vi "Ball Align(SubVI).vi"(0 "Align X - t, Y - f":bool, 3 "x is in range":bool, 4 "y is in range":bool, 5 "L_PWM":dbl, 6 "R_PWM":dbl, 7 "curX":dbl, 8 "defY":dbl, 9 "curY":dbl, 14 "defX":dbl, 16 "Range":dbl) -> (13 "x_is_in_range":bool, 15 "y_is_in_range":bool, 20 "Align_X-t,Y-f":bool, 21 "Boolean 4":bool, 23 "Boolean":bool, 24 "Boolean 3":bool, 25 "Boolean 2":bool, 26 "L_PWM out":dbl, 27 "R_PWM out":dbl)   [LabVIEW 2017]
panel:
  in  "extra power":dbl format="%#_13g"
  in  "range for boost":dbl
  out "offset":bool
  in  "M_offsetX":dbl
  in  "M_defY":dbl
  # "IN"
  # "OUT"
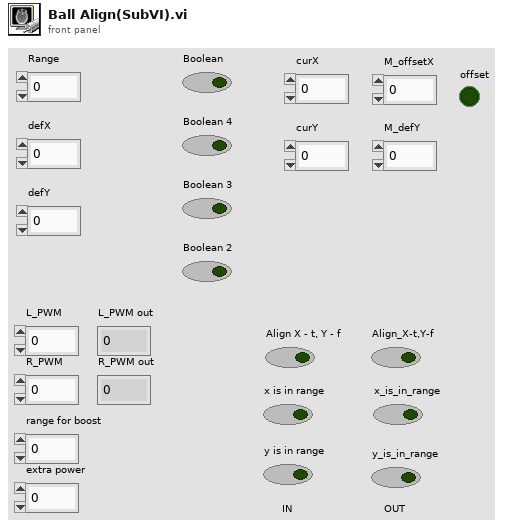
[diagram p1: front panel]
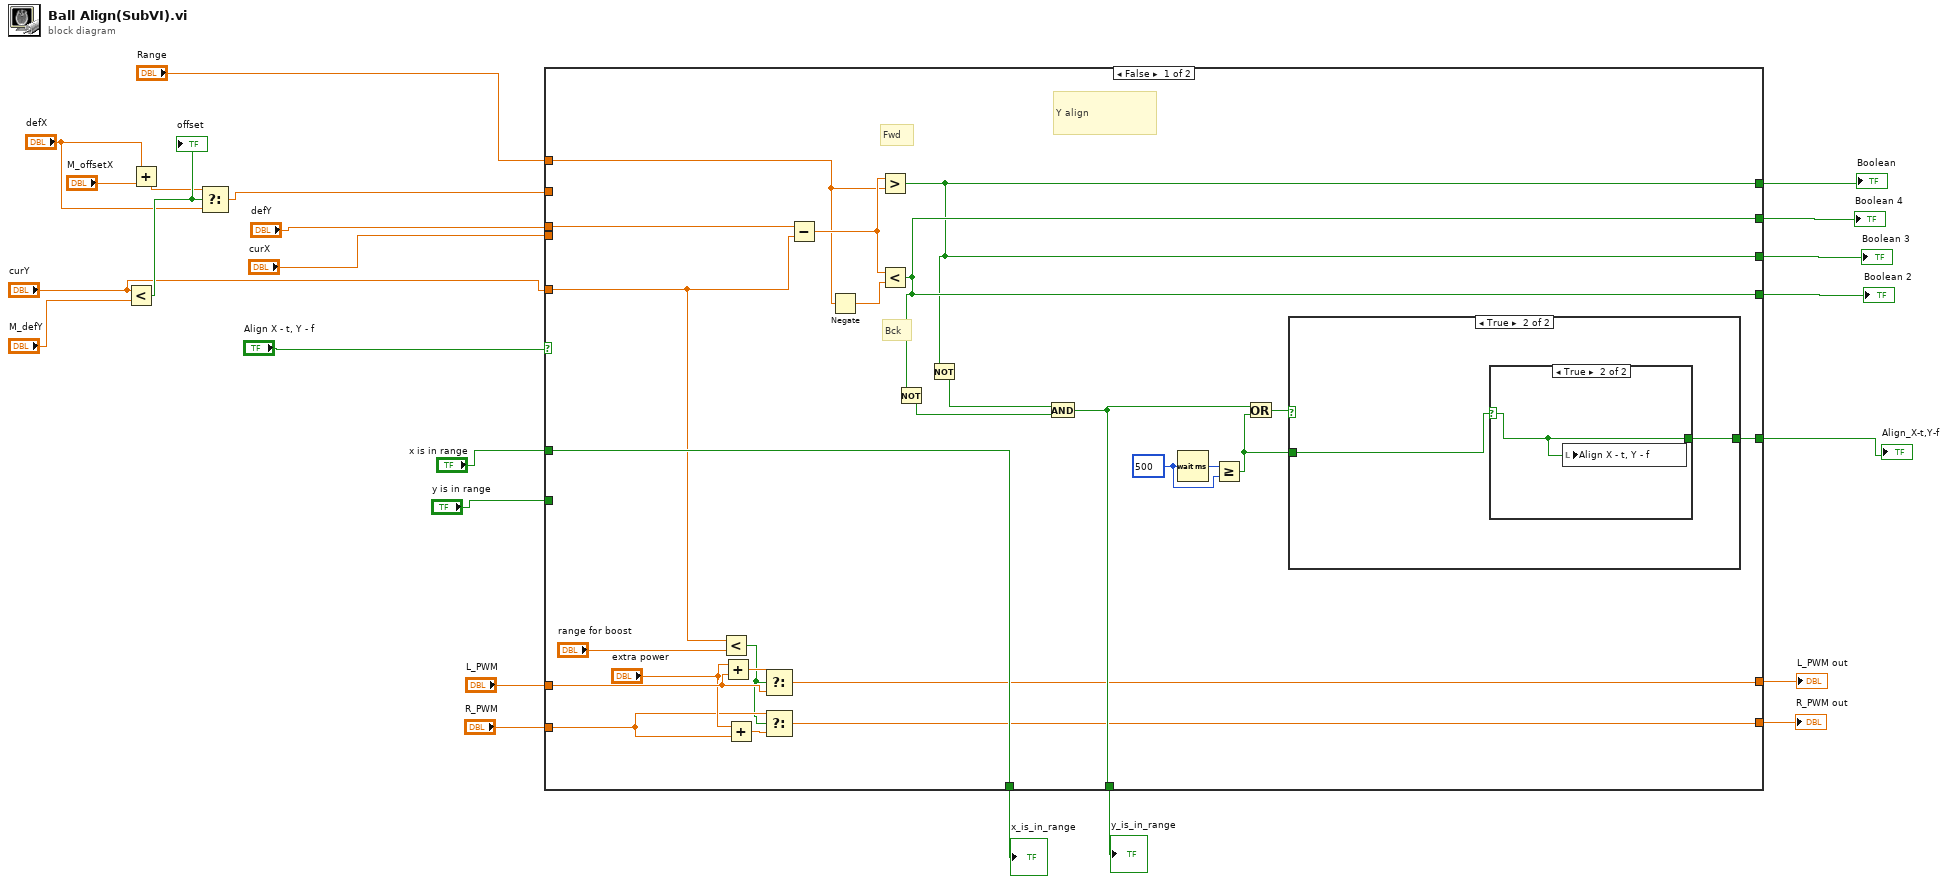
[diagram p0: block diagram]
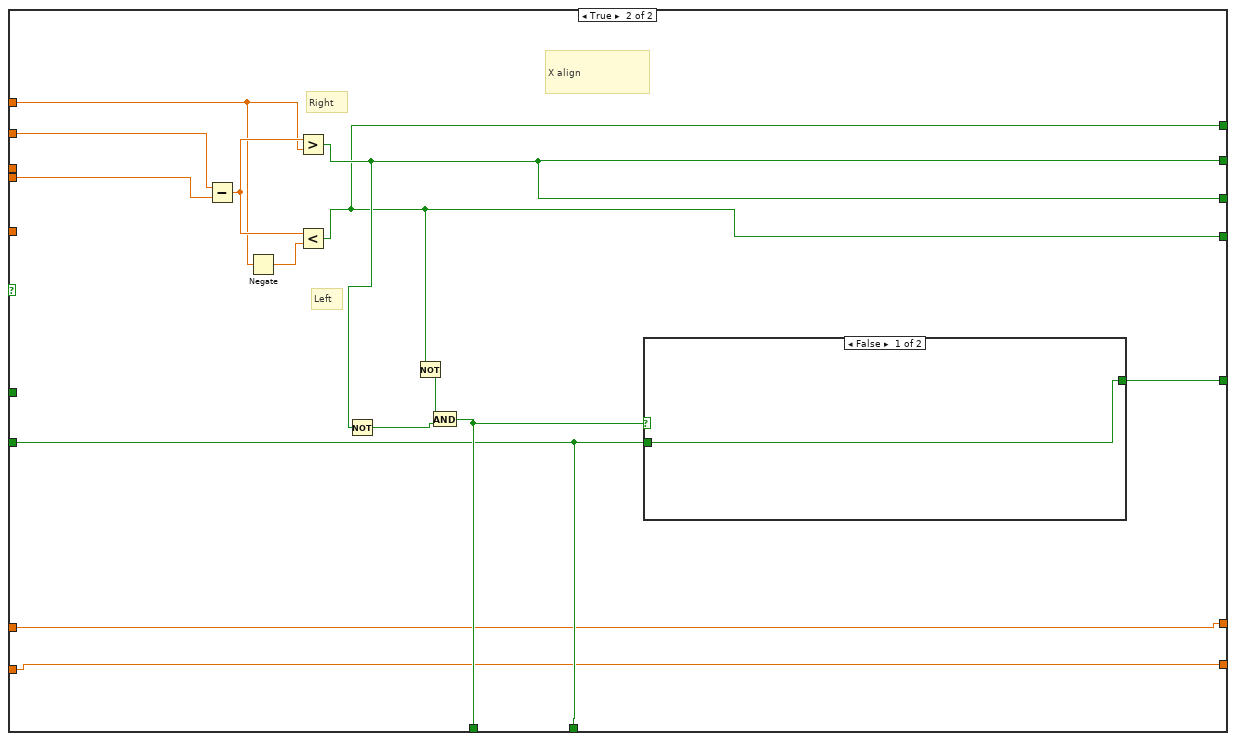
[diagram p4: hidden frame]
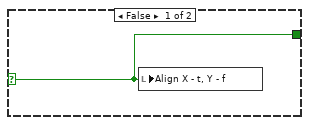
[diagram p6: hidden frame]
diagram:
  n1 = Less?(x="curY", y="M_defY") -> (x < y?=w13:bool)
  "offset" <- w13
  n2 = Add(x="defX", y="M_offsetX") -> (x+y=w11:dbl)
  n3 = Select(t=w11, s=w13, f="defX") -> (s? t:f=w9:dbl)
  n4 = case shown="False" "Align X - t, Y - f" {
    tunnel: w9 -> [_ w64]
    tunnel: "curX" -> [_ w63]
    tunnel: "Range" -> [w46 w62]
    tunnel: "defY" -> [w47 _]
    tunnel: "curY" -> [w34 _]
    tunnel: [w45 w58] -> w19
    tunnel: [w36 w61] -> w20
    tunnel: [w44 w60] -> w21
    tunnel: [w43 w60] -> w22
    tunnel: [w44 w59] -> w23
    tunnel: [w43 w59] -> w24
    tunnel: "x is in range" -> [w36 _]
    tunnel: "y is in range" -> [_ w58]
    tunnel: [w35 w57] -> w5
    tunnel: "L_PWM" -> [w31 w55]
    tunnel: "R_PWM" -> [w28 w56]
    tunnel: [w27 w55] -> w2
    tunnel: [w26 w56] -> w1
    frame False {
      w39 = u32 500 ("milliseconds to wait")
      # "Bck"
      # "Fwd"
      # "Y align"
      n5 = Less?(x=w34, y="range for boost") -> (x < y?=w25:bool)
      n6 = Add(x="extra power", y=w31) -> (x+y=w32:dbl)
      n7 = Add(x="extra power", y=w28) -> (x+y=w30:dbl)
      n8 = Select(t=w32, s=w25, f=w31) -> (s? t:f=w27:dbl)
      n9 = Select(t=w28, s=w25, f=w30) -> (s? t:f=w26:dbl)
      n10 = Subtract(x=w47, y=w34) -> (x-y=w49:dbl)
      n11 = Negate(x=w46) -> (-x=w48:dbl)
      n12 = Greater?(x=w49, y=w46) -> (0:w43:bool)
      n13 = Less?(x=w49, y=w48) -> (x < y?=w44:bool)
      n14 = Not(x=w44) -> (.not. x?=w41:bool)
      n15 = Not(x=w43) -> (.not. x?=w42:bool)
      n16 = And(x=w42, y=w41) -> (x .and. y?=w45:bool)
      n17 = Wait (ms)(milliseconds to wait=w39) -> (millisecond timer value=w40:u32)
      n18 = Greater Or Equal?(x=w40, y=w39) -> (x >= y?=w37:bool)
      n19 = Or(x=w45, y=w37) -> (x .or. y?=w38:bool)
      n20 = case shown="True" w38 {
        selector: w38 -> [w50 _]
        tunnel: w37 -> [_ w52]
        tunnel: [w50 w51] -> w35
        frame False {
        }
        frame True {
          n21 = case shown="True" w52 {
            selector: w52 -> [w53 w54]
            tunnel: [w53 w54] -> w51
            frame False {
            }
            frame True {
              n22 = local write "Align X - t, Y - f"(w54) -> ()
            }
          }
        }
      }
    }
    frame True {
      # "X align"
      # "Right"
      # "Left"
      n23 = Subtract(x=w64, y=w63) -> (x-y=w68:dbl)
      n24 = Negate(x=w62) -> (-x=w67:dbl)
      n25 = Greater?(x=w68, y=w62) -> (0:w60:bool)
      n26 = Less?(x=w68, y=w67) -> (x < y?=w59:bool)
      n27 = Not(x=w60) -> (.not. x?=w65:bool)
      n28 = Not(x=w59) -> (.not. x?=w66:bool)
      n29 = And(x=w66, y=w65) -> (x .and. y?=w61:bool)
      n30 = case shown="False" w61 {
        tunnel: w58 -> [w69 w71]
        tunnel: [w69 w70] -> w57
        frame False {
        }
        frame True {
          n31 = case shown="True" w71 {
            selector: w71 -> [w72 w73]
            tunnel: [w72 w73] -> w70
            frame False {
              n32 = local write "Align X - t, Y - f"(w72) -> ()
            }
            frame True {
            }
          }
        }
      }
    }
  }
  "Boolean" <- w24
  "Boolean 2" <- w23
  "Boolean 3" <- w22
  "Boolean 4" <- w21
  "x_is_in_range" <- w20
  "y_is_in_range" <- w19
  "Align_X-t,Y-f" <- w5
  "L_PWM out" <- w2
  "R_PWM out" <- w1
